vi "LZW decode.vi"(0 "data":string, 1 "expected data size":i32=10000, 5 "NumberOfStartBits":u8, 11 "error in (no error)":errorcluster) -> (6 "decoded data":i32[](array[numeric]), 15 "error out":errorcluster)   [LabVIEW 2011, in "Gif Image.lvclass"]
uses:
  Gif Image.lvclass
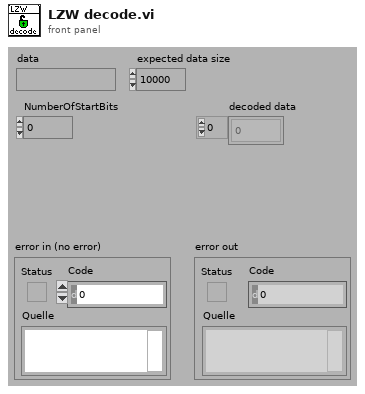
[diagram p1: front panel]
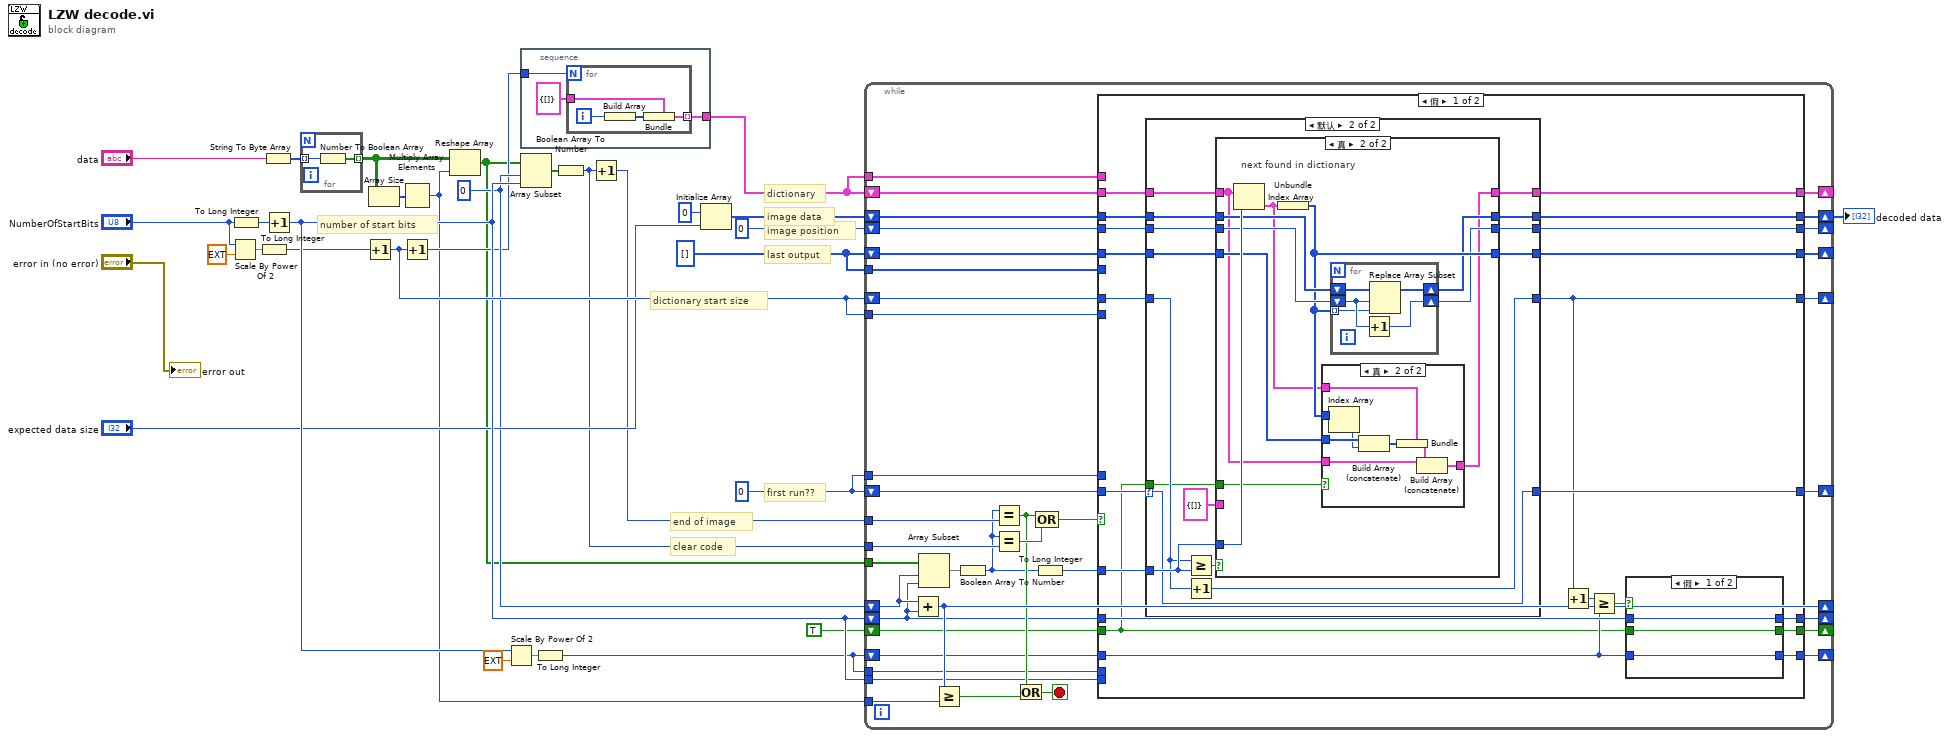
[diagram p0: block diagram]
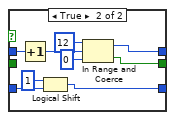
[diagram p2: hidden frame]
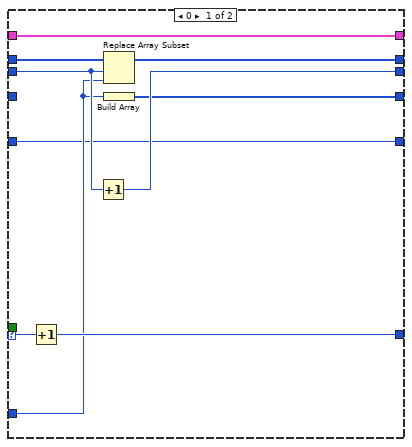
[diagram p3: hidden frame]
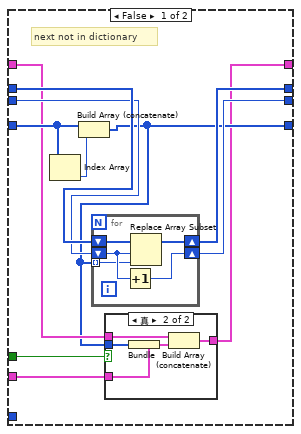
[diagram p4: hidden frame]
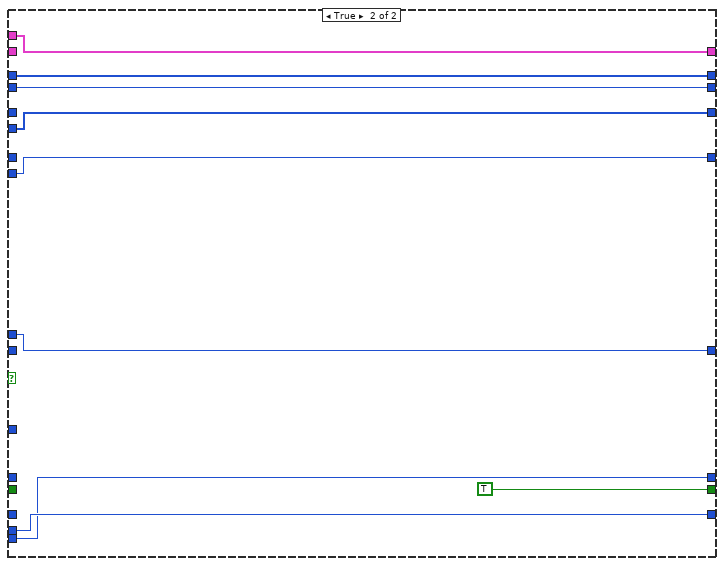
[diagram p7: hidden frame]
diagram:
  w29 = 0
  w22 = i32[] []
  w15 = 0 ("length")
  # "first run??"
  # "last output"
  # "dictionary"
  # "image position"
  # "image data"
  # "dictionary start size"
  # "end of image"
  # "clear code"
  # "number of start bits"
  n1 = Scale By Power Of 2(n="NumberOfStartBits", x=ext 1.0) -> (x*2^n=w6:ext)
  n2 = To Long Integer(number="NumberOfStartBits") -> (32bit integer=w8:i32)
  n3 = To Long Integer(number=w6) -> (32bit integer=w26:i32)
  n4 = String To Byte Array(string="data") -> (unsigned byte array=w13:u8[])
  n5 = Increment(x=w8) -> (x+1=w28:i32)
  n6 = for {
    tunnel: w13 -> [w33] mode=indexing
    tunnel: [w32] -> w3 mode=indexing
    n7 = Number To Boolean Array(number=w33) -> (Boolean array=w32:bool[])
  }
  n8 = Increment(x=w26) -> (x+1=w31:i32)
  n9 = Array Size(array=w3) -> (size(s)=w4:i32[])
  n10 = Multiply Array Elements(1:w4) -> (0:w9:i32)
  n11 = Increment(x=w31) -> (x+1=w14:i32)
  n12 = Reshape Array(w3, w9) -> (w11:bool[])
  n13 = Scale By Power Of 2(n=w28, x=ext 1.0) -> (x*2^n=w24:ext)
  n14 = stacked-sequence {
    tunnel: [w35] -> w23
    tunnel: w14 -> [w34]
    frame #0 {
      n15 = for {
        N: w34 -> [_]
        tunnel: cluster{i32[]} {[]} -> [w38]
        tunnel: [w37] -> w35 mode=indexing
        i -> [w40]
        n16 = Build Array(w40) -> (w39:i32[])
        n17 = Bundle(cluster=w38, w39) -> (w37:cluster{i32[]})
      }
    }
  }
  n18 = Array Subset(array=w11, index=w15, length=w28) -> (w10:bool[])
  n19 = To Long Integer(number=w24) -> (32bit integer=w27:i32)
  n20 = Boolean Array To Number(Boolean array=w10) -> (number=w16:u32)
  n21 = Increment(x=w16) -> (x+1=w17:u32)
  n22 = Initialize Array(0 ("element"), "expected data size") -> (w20:i32[])
  n23 = while {
    tunnel: w11 -> [w77]
    shift-right: [w52] -> _
    shift-left: w28 -> [w54]
    shift-right: [w75] -> _
    shift-left: w15 -> [w76]
    tunnel: w9 -> [w74]
    tunnel: w16 -> [w73]
    tunnel: w17 -> [w72]
    shift-right: [w55] -> _
    shift-left: w31 -> [w56]
    shift-right: [w64] -> w30
    shift-left: w20 -> [w60]
    shift-right: [w63] -> _
    shift-left: 0 ("element") -> [w58]
    shift-right: [w66] -> _
    shift-left: w23 -> [w59]
    shift-right: [w61] -> _
    shift-left: w22 -> [w57]
    tunnel: w23 -> [w65]
    tunnel: w22 -> [w62]
    shift-right: [w51] -> _
    shift-left: w27 -> [w53]
    tunnel: w27 -> [w50]
    tunnel: w28 -> [w49]
    shift-right: [w47] -> _
    shift-left: w29 -> [w48]
    tunnel: w29 -> [w46]
    tunnel: w31 -> [w43]
    shift-right: [w42] -> _
    shift-left: TRUE -> [w41]
    stop <- w67 stop-if-true
    n24 = Add(x=w76, y=w54) -> (x+y=w75:i32)
    n25 = Array Subset(array=w77, index=w76, length=w54) -> (w78:bool[])
    n26 = Greater Or Equal?(x=w75, y=w74) -> (x >= y?=w68:bool)
    n27 = Boolean Array To Number(Boolean array=w78) -> (number=w45:u32)
    n28 = Equal?(x=w45, y=w72) -> (x = y?=w69:bool)
    n29 = Equal?(x=w45, y=w73) -> (x = y?=w71:bool)
    n30 = Or(x=w69, y=w68) -> (x .or. y?=w67:bool)
    n31 = To Long Integer(number=w45) -> (32bit integer=w44:i32)
    n32 = Compound Arithmetic op=OR(w69, w71) -> (w70:bool)
    n33 = case shown="假" w70 {
      tunnel: w44 -> [w95 _]
      tunnel: [w91 w192] -> w66
      tunnel: w65 -> [_ w192]
      tunnel: [w93 w186] -> w64
      tunnel: [w94 w185] -> w63
      tunnel: w62 -> [_ w191]
      tunnel: [w90 w191] -> w61
      tunnel: w60 -> [w97 w186]
      tunnel: w59 -> [w92 _]
      tunnel: w58 -> [w96 w185]
      tunnel: w57 -> [w81 _]
      tunnel: w56 -> [w89 _]
      tunnel: [w88 w187] -> w55
      tunnel: w54 -> [w85 _]
      tunnel: w53 -> [w82 _]
      tunnel: [w84 w189] -> w52
      tunnel: [w83 w190] -> w51
      tunnel: w50 -> [_ w190]
      tunnel: w49 -> [_ w189]
      tunnel: w48 -> [w99 _]
      tunnel: [w98 w188] -> w47
      tunnel: w46 -> [_ w188]
      tunnel: w43 -> [_ w187]
      tunnel: [w80 TRUE] -> w42
      tunnel: w41 -> [w79 _]
      frame False {
        n34 = case shown="默认" w99 {
          selector: w99 -> [w121 w123]
          tunnel: [w120 w123] -> w98
          tunnel: w97 -> [w119 w134]
          tunnel: w96 -> [w118 w132]
          tunnel: w95 -> [w114 w130]
          tunnel: [w117 w127] -> w94
          tunnel: [w116 w128] -> w93
          tunnel: w92 -> [w115 w131]
          tunnel: [w115 w126] -> w91
          tunnel: [w113 w129] -> w90
          tunnel: [w112 w136] -> w88
          tunnel: w89 -> [w112 w125]
          tunnel: w81 -> [_ w133]
          tunnel: w79 -> [_ w122]
          frame 0 {
            n35 = Increment(x=w121) -> (x+1=w120:i32)
            n36 = Increment(x=w118) -> (x+1=w117:i32)
            n37 = Replace Array Subset(array=w119, new element=w114, index=w118) -> (w116:i32[])
            n38 = Build Array(w114) -> (w113:i32[])
          }
          frame Default {
            n39 = Greater Or Equal?(x=w125, y=w130) -> (x >= y?=w135:bool)
            n40 = Increment(x=w125) -> (x+1=w136:i32)
            n41 = case shown="真" w135 {
              tunnel: w134 -> [w145 w168]
              tunnel: w133 -> [w147 w163]
              tunnel: w132 -> [w144 w167]
              tunnel: w131 -> [w141 w161]
              tunnel: w130 -> [_ w169]
              tunnel: [w139 w166] -> w129
              tunnel: [w143 w165] -> w128
              tunnel: [w142 w164] -> w127
              tunnel: cluster{i32[]} {[]} -> [w140 _]
              tunnel: [w138 w160] -> w126
              tunnel: w122 -> [w137 w159]
              frame False {
                # "next not in dictionary"
                n42 = Index Array(array=w147) -> (element=w146:i32)  [unwired: 1 in]
                n43 = Build Array (concatenate)(w147, w146) -> (w139:i32[])
                n44 = for {
                  shift-right: [w157] -> w143
                  shift-left: w145 -> [w158]
                  shift-right: [w155] -> w142
                  shift-left: w144 -> [w156]
                  tunnel: w139 -> [w154] mode=indexing
                  n45 = Increment(x=w156) -> (x+1=w155:i32)
                  n46 = Replace Array Subset(array=w158, new element=w154, index=w156) -> (w157:i32[])
                }
                n47 = case shown="真" w137 {
                  tunnel: w141 -> [w148 w153]
                  tunnel: w140 -> [_ w152]
                  tunnel: w139 -> [_ w151]
                  tunnel: [w148 w150] -> w138
                  frame False {
                  }
                  frame True {
                    n48 = Bundle(cluster=w152, w151) -> (w149:cluster{i32[]})
                    n49 = Build Array (concatenate)(w153, w149) -> (w150:cluster{i32[]}[])
                  }
                }
              }
              frame True {
                # "next found in dictionary"
                n50 = Index Array(array=w161, index=w169) -> (element=w162:cluster{i32[]})
                n51 = Unbundle(w162) -> (w166:i32[])
                n52 = case shown="真" w159 {
                  tunnel: w166 -> [_ w178]
                  tunnel: w163 -> [_ w177]
                  tunnel: w162 -> [_ w175]
                  tunnel: w161 -> [w170 w173]
                  tunnel: [w170 w171] -> w160
                  frame False {
                  }
                  frame True {
                    n53 = Index Array(array=w178) -> (element=w176:i32)  [unwired: 1 in]
                    n54 = Build Array (concatenate)(w177, w176) -> (w174:i32[])
                    n55 = Bundle(cluster=w175, w174) -> (w172:cluster{i32[]})
                    n56 = Build Array (concatenate)(w173, w172) -> (w171:cluster{i32[]}[])
                  }
                }
                n57 = for {
                  shift-right: [w182] -> w165
                  shift-left: w168 -> [w183]
                  shift-right: [w180] -> w164
                  shift-left: w167 -> [w181]
                  tunnel: w166 -> [w179] mode=indexing
                  n58 = Increment(x=w181) -> (x+1=w180:i32)
                  n59 = Replace Array Subset(array=w183, new element=w179, index=w181) -> (w182:i32[])
                }
              }
            }
          }
        }
        n60 = Increment(x=w88) -> (x+1=w87:i32)
        n61 = Greater Or Equal?(x=w87, y=w82) -> (x >= y?=w86:bool)
        n62 = case shown="假" w86 {
          tunnel: w85 -> [w102 w111]
          tunnel: [w102 w104] -> w84
          tunnel: [w101 w108] -> w83
          tunnel: w82 -> [w101 w110]
          tunnel: [w100 w103] -> w80
          tunnel: w79 -> [w100 _]
          frame False {
          }
          frame True {
            n63 = Increment(x=w111) -> (x+1=w105:i32)
            n64 = Logical Shift(y=1, x=w110) -> (x << y=w108:i32)
            n65 = In Range and Coerce(upper limit=12, x=w105, lower limit=0) -> (coerced(x)=w104:i32, In Range?=w103:bool)
          }
        }
      }
      frame True {
      }
    }
  }
  "decoded data" <- w30
  "error out" <- "error in (no error)"
